vi "Configure Voltage and Current Limit.vi"(7 "Settle (0 mS)":u32, 8 "error":errorcluster, 9 "Current Limit":dbl format="%.4f", 10 "Voltage Limit":dbl format="%.4f", 11 "VISA in":refnum<visa-resource-name>) -> (0 "error out":errorcluster, 3 "VISA out":refnum<visa-resource-name>)   [LabVIEW 2023, in "TDK20-38 API.lvlib"]
uses:
  TDK20-38 API.lvlib
  LabVIEW - Drivers/Genesys Drivers/LAN/TDK-Lambda GEN LAN Series.lvlib
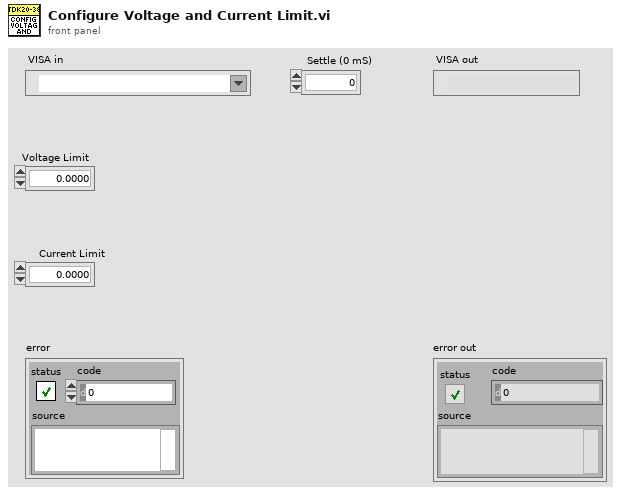
[diagram p1: front panel]
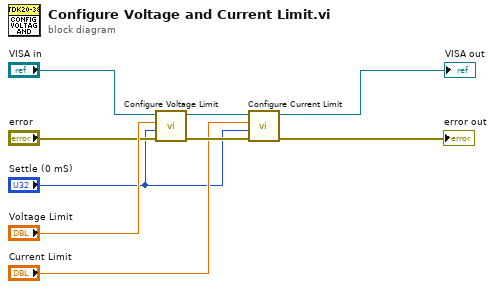
[diagram p0: block diagram]
diagram:
  n1 = call "Configure Voltage Limit.vi"("error"="error", "Settle (0 mS)"="Settle (0 mS)", "Voltage Limit"="Voltage Limit", "VISA"="VISA in") -> ("error out"=w4:errorcluster, "VISA out"=w8:refnum<visa-resource-name>)  [unwired: 6 in]
  n2 = call "Configure Current Limit.vi"("error"=w4, "Settle (0 mS)"="Settle (0 mS)", "Current Limit"="Current Limit", "VISA"=w8) -> ("error out"=→"error out":errorcluster, "VISA out"=→"VISA out":refnum<visa-resource-name>)  [unwired: 6 in]
